vi "Compress Single File.vi"(8 "error in (no error)":errorcluster, 9 "Internal Name":path, 10 "Source File Path":path, 11 "Zip File Path":path) -> (0 "error out":errorcluster, 1 "Standard Output":string, 3 "dup Zip File Path":path)   [LabVIEW 2019, in "Command-Line Zip.lvlib"]
uses:
  Command-Line Zip.lvlib
  <userlib>/_OpenG.lib/file/file.llb/Compare Two Paths - Scalar__ogtk.vi
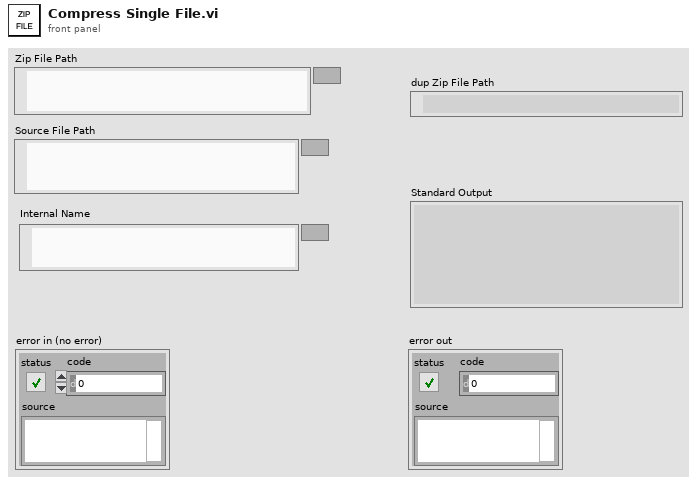
[diagram p1: front panel]
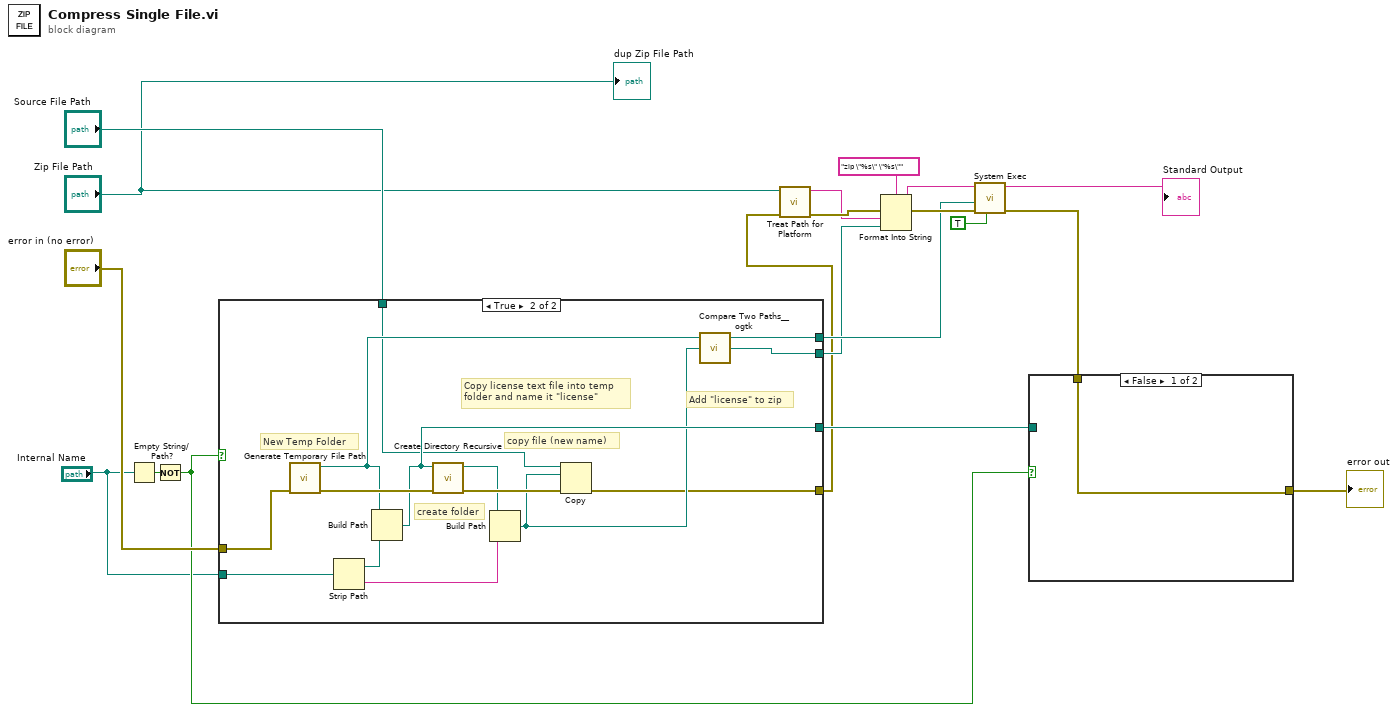
[diagram p0: block diagram]
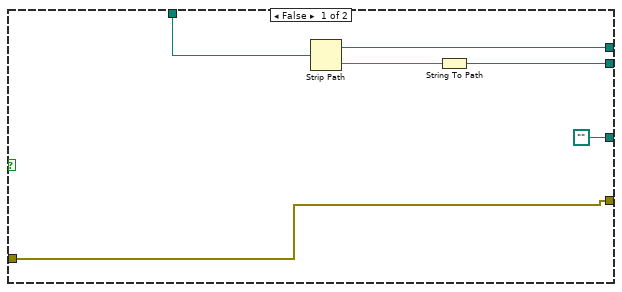
[diagram p2: hidden frame]
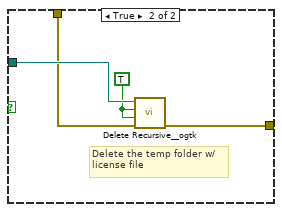
[diagram p3: hidden frame]
diagram:
  n1 = Empty String/Path?(string/path="Internal Name") -> (empty?=w4:bool)
  n2 = Not(x=w4) -> (.not. x?=w3:bool)
  n3 = case shown="True" w3 {
    tunnel: [w24 w39] -> w12
    tunnel: [w22 w38] -> w11
    tunnel: [path "" w34] -> w10
    tunnel: "Source File Path" -> [w25 w30]
    tunnel: "error in (no error)" -> [w20 w29]
    tunnel: "Internal Name" -> [_ w27]
    tunnel: [w20 w26] -> w1
    frame False {
      n4 = Strip Path(path=w25) -> (stripped path=w24:path, name=w23:string)
      n5 = String To Path(string=w23) -> (path=w22:path)
    }
    frame True {
      # "New Temp Folder"
      # "copy file (new name)"
      # "create folder"
      # "Add \"license\" to zip"
      # "Copy license text file into temp folder and name it \"license\""
      n6 = call <vilib>:"Generate Temporary File Path.vi"("error in (no error)"=w29) -> ("error out"=w37:errorcluster, "Unique Temporary File Path"=w31:path)  [unwired: 9 in]
      n7 = Strip Path(path=w27) -> (stripped path=w33:path, name=w32:string)
      n8 = Build Path(base path=w31, name or relative path=w33) -> (appended path=w34:path)
      n9 = call <vilib>:"Create Directory Recursive.vi"("error in (no error)"=w37, "directory"=w34) -> ("error out"=w36:errorcluster, "directory copy"=w35:path)  [unwired: 3 in, 1 out]
      n10 = Build Path(base path=w35, name or relative path=w32) -> (appended path=w28:path)
      n11 = Copy(8:w36, 10:w28, 11:w30) -> (0:w26:errorcluster)  [unwired: 2 in, 2 out]
      n12 = call-poly <userlib>:"Compare Two Paths__ogtk.vi"("path2"=w28, "path1"=w31) -> ("relative path from 1 to 2"=w38:path, "common path"=w39:path)  [unwired: 1 in, 1 out]
    }
  }
  n13 = call "Treat Path for Platform.vi"("error in (no error)"=w1, "File Path"="Zip File Path") -> ("error out"=w19:errorcluster, "Path for CLI"=w18:string)  [unwired: 8 in]
  n14 = Format Into String(format string="zip \"%s\" \"%s\"" ("command line"), error in=w19, w18, w11) -> (resulting string=w15:string, error out=w16:errorcluster)  [unwired: 1 in]
  n15 = call <vilib>:"System Exec.vi"("run minimized? (F)"=TRUE, "error in (no error)"=w16, "working directory"=w12, "command line"=w15) -> ("error out"=w7:errorcluster, "standard output"=→"Standard Output":string)  [unwired: 4 in, 2 out]
  n16 = case shown="False" w3 {
    tunnel: w10 -> [_ w44]
    tunnel: w7 -> [w40 w43]
    tunnel: [w40 w42] -> w6
    frame False {
    }
    frame True {
      w41 = TRUE ("entire hierarchy (F)")
      # "Delete the temp folder w/\nlicense file"
      n17 = call <userlib>:"Delete Recursive__ogtk.vi"("error in (no error)"=w43, "Ignore Read-Only? (FALSE)"=w41, "Recursive? (FALSE)"=w41, "Path"=w44) -> ("error out"=w42:errorcluster)  [unwired: 6 in, 1 out]
    }
  }
  "error out" <- w6
  "dup Zip File Path" <- "Zip File Path"
